vi "Init.vi"(8 "error in (no error)":errorcluster, 11 "BetterTreeHandle in":refnum<class "BetterTreeHandle.lvclass">) -> (0 "error out":errorcluster, 3 "BetterTreeHandle out":refnum<class "BetterTreeHandle.lvclass">)   [LabVIEW 2020, in "BetterDragAndDrop.lvlib" / "BetterTreeHandle.lvclass"]
uses:
  BetterTreeHandle.lvclass
  C:/DSCE code/Open-source/betterdraganddrop_GIT/Source/Classes/BetterHandle/BetterHandle.lvclass
  BetterTreeHandle.lvclass/BetterTreeHandle.ctl
  BetterHandle/Pixel Constants.ctl
  BetterHandle/BetterHandle.lvclass/BetterHandle.ctl
  BetterHandle/Write Constant Sizes.vi
  BetterHandle/BetterHandle.lvclass
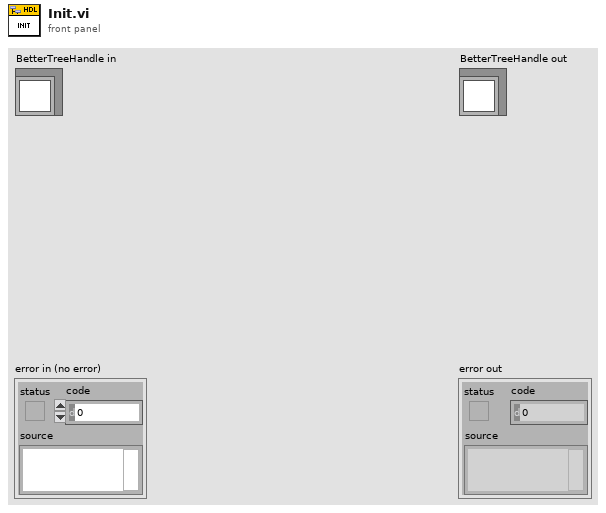
[diagram p1: front panel]
types:
  T1 = typedef "BetterDragAndDrop.lvlib/BetterHandle.lvclass/Pixel Constants.ctl" = cluster{"Row Header height":i32, "Row height":i32, "Column Header Offset":i32}
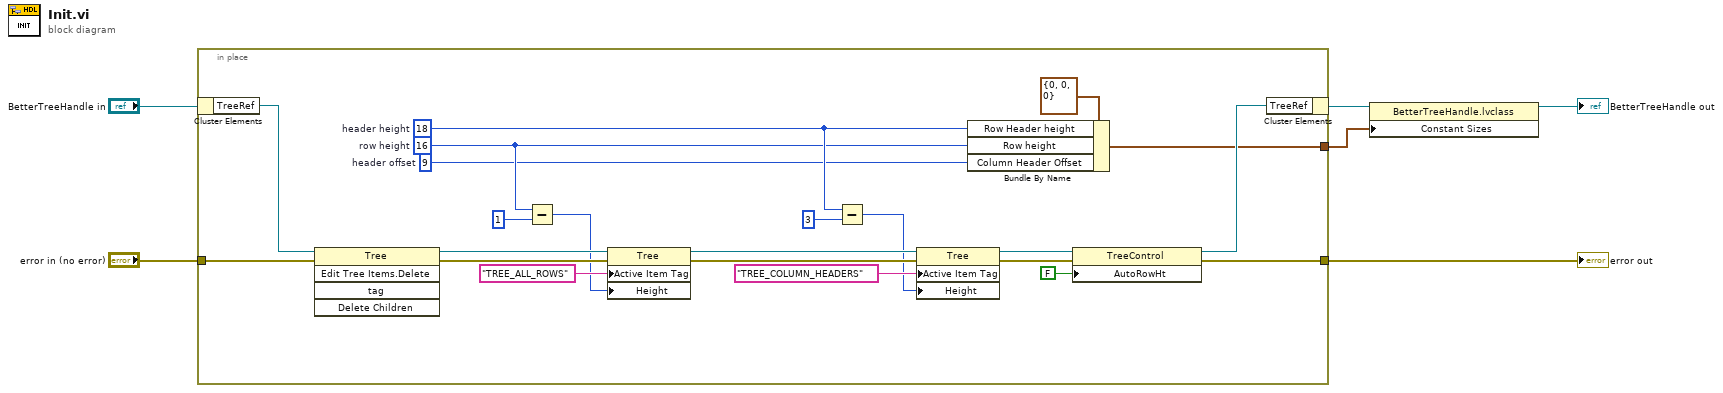
[diagram p0: block diagram]
diagram:
  n1 = in-place {
    in-place-border: "error in (no error)" -> [w28]
    in-place-border: [w13] -> w4
    in-place-border: [w7] -> w1
    w8 = 9  # header offset
    w9 = 16  # row height
    w10 = 18  # header height
    n2 = in-place-cluster #1("BetterTreeHandle in") -> ("TreeRef"=w27:refnum<vi>)
    n3 = invoke class="Tree" method="Edit Tree Items.Delete"(reference=w27, error in=w28) -> (reference out=w23:refnum<vi>, error out=w22:errorcluster)  [unwired: 3 in, 3 out]
    n4 = Subtract(x=w9, y=1) -> (x-y=w19:i32)
    n5 = property class="Tree"(reference=w23, error in=w22, "Active Item Tag"="TREE_ALL_ROWS" ("Active Item:Tag"), "Height"=w19) -> (reference out=w24:refnum<vi>, error out=w21:errorcluster)
    n6 = Subtract(x=w10, y=3) -> (x-y=w17:i32)
    n7 = property class="Tree"(reference=w24, error in=w21, "Active Item Tag"="TREE_COLUMN_HEADERS" ("Active Item:Tag"), "Height"=w17) -> (reference out=w12:refnum<vi>, error out=w16:errorcluster)
    n8 = Bundle By Name(cluster=T1 {"Row Header height"=0, "Row height"=0, "Column Header Offset"=0} ("Constant Sizes"), "Row Header height"=w10, "Row height"=w9, "Column Header Offset"=w8) -> (w7:T1)
    n9 = property class="TreeControl"(reference=w12, error in=w16, "AutoRowHt"=FALSE ("Autosizing Row Height")) -> (reference out=w14:refnum<vi>, error out=w13:errorcluster)
    n10 = in-place-cluster #1("TreeRef"=w14) -> (w3:refnum<class "BetterTreeHandle.lvclass">)
  }
  "error out" <- w4
  n11 = property class="BetterTreeHandle.lvclass"(reference=w3, "Constant Sizes"=w1) -> (reference out=→"BetterTreeHandle out":refnum<class "BetterTreeHandle.lvclass">)  [unwired: 1 in, 1 out]
